vi "SigGen.vi"(0 "Amp":dbl, 1 "Freq":dbl, 2 "Offset":dbl, 3 "Timer":dbl, 4 "Type":dbl) -> (5 "Output":dbl)   [LabVIEW 2017]
uses:
  <vilib>/gmath/NI_Gmath.lvlib
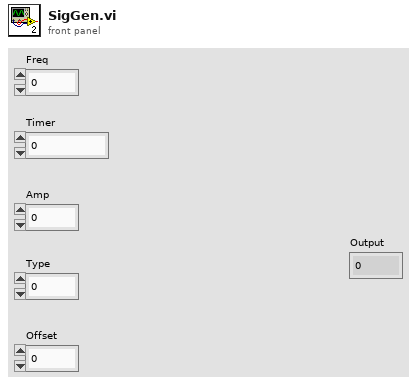
[diagram p1: front panel]
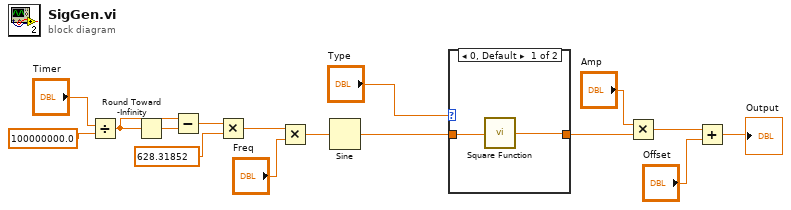
[diagram p0: block diagram]
diagram:
  n1 = Divide(x="Timer", y=100000000.0) -> (x/y=w14:dbl)
  n2 = Round Toward -Infinity(1:w14) -> (0:w15:dbl)
  n3 = Subtract(x=w14, y=w15) -> (x-y=w13:dbl)
  n4 = Multiply(x=w13, y=628.31852) -> (x*y=w11:dbl)
  n5 = Multiply(x=w11, y="Freq") -> (x*y=w9:dbl)
  n6 = Sine(x=w9) -> (sin(x)=w2:dbl)
  n7 = case shown="0, Default" "Type" {
    tunnel: w2 -> [w18 w19]
    tunnel: [w17 w19] -> w5
    frame 0, Default {
      n8 = call <vilib>:"Square Function.vi"("x"=w18) -> ("square(x)"=w17:dbl)
    }
    frame 1 {
    }
  }
  n9 = Multiply(x="Amp", y=w5) -> (x*y=w4:dbl)
  n10 = Add(x=w4, y="Offset") -> (x+y=→"Output":dbl)
